vi "Actor Core.vi"(8 "error in (no error)":errorcluster, 11 "Websocket Client Handler in":refnum<class "Websocket Client Handler.lvclass">) -> (0 "error out":errorcluster, 3 "Mediated Asynchronous Actor out":refnum<class "Websocket Client Handler.lvclass">)   [LabVIEW 2016, in "Stream Mediator.lvlib" / "Websocket Client Handler.lvclass"]
doc: "--\nCopyright © 2017 Composed SystemsI All rights reserved.\n\nAuthor: Jon McBee <jon.mcbee@composed.io>\n\nThis library is provided \"AS IS\" ,WITHOUT WARRANTIES OR\nCONDITIONS OF ANY KIND, either express or implied.\n\nComposed Systems -- composed.io\n\nStream 0.0.1.1\nJon McBee - Composed Systems\nCopyright (c) 2017, Composed Systems"
uses:
  <userlib>/Composed Systems/Stream/Mediator/Classes/Websocket Client Handler Actor/Websocket Client Handler/Websocket Client Handler.lvclass
  C:/Program Files (x86)/National Instruments/LabVIEW 2016/user.lib/Composed Systems/Stream/Mediator/Classes/Mediated Asynchronous Actor/Mediated Asynchronous Actor.lvclass
  C:/Program Files (x86)/National Instruments/LabVIEW 2016/user.lib/Composed Systems/Stream/Mediator/Classes/Mediated Actor/Mediated Actor.lvclass
  <userlib>/Composed Systems/Stream/Mediator/Classes/Message Transport Event/Message Transport Event.lvclass
  C:/Program Files (x86)/National Instruments/LabVIEW 2016/user.lib/Composed Systems/Stream/Mediator/Classes/Message Transport Interface/Message Transport Interface.lvclass
  <userlib>/Composed Systems/Stream/Mediator/Classes/Mediated Asynchronous Actor/Mediated Asynchronous Actor.lvclass
  <userlib>/Composed Systems/Stream/Mediator/Classes/Message Broker Interface/Message Broker Interface.lvclass
  <userlib>/Composed Systems/Stream/Mediator/Classes/Websocket Client Handler Actor/Websocket Client Handler Msgs/Write Msg/Write Msg.lvclass
  <userlib>/Composed Systems/Stream/Mediator/Classes/Mediated Actor/Mediated Actor.lvclass
  <userlib>/Composed Systems/Stream/Mediator/Classes/Websocket Client Handler Actor/Websocket Client Handler Msgs/Read Msg/Read Msg.lvclass
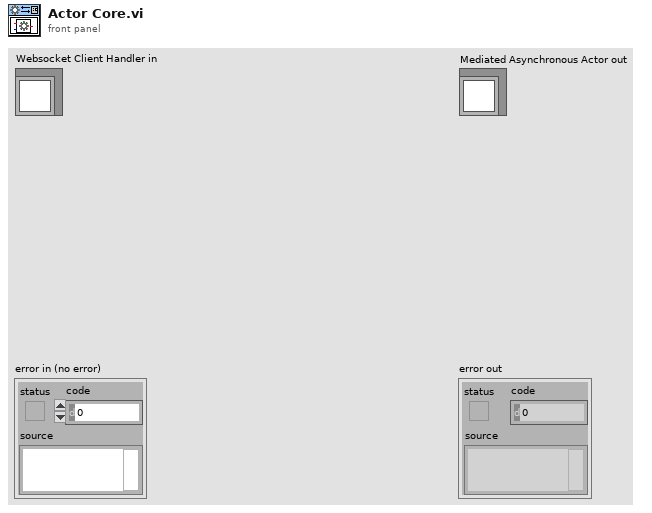
[diagram p1: front panel]
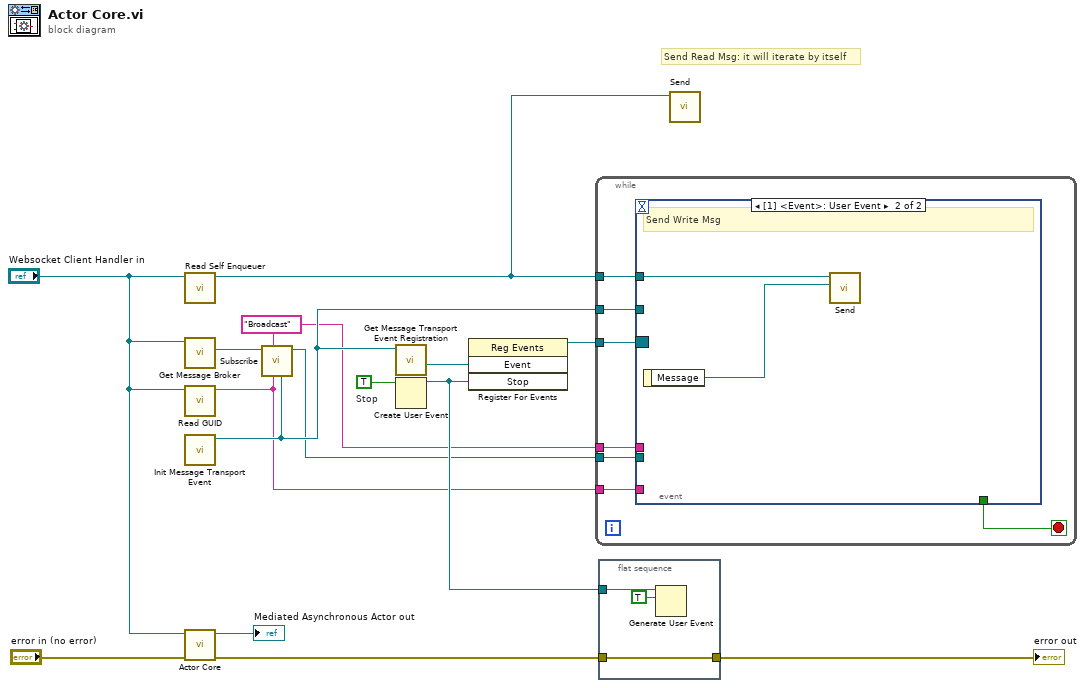
[diagram p0: block diagram]
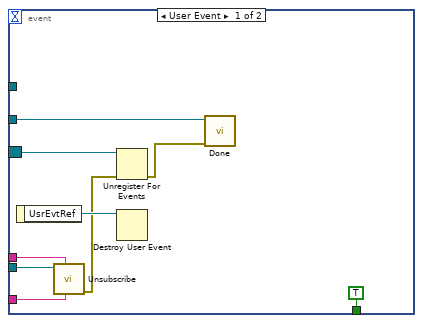
[diagram p2: hidden frame]
diagram:
  w2 = "Broadcast" ("Topic Name")
  w14 = TRUE  # Stop
  # "Send Read Msg: it will iterate by itself"
  n1 = call <userlib>:"Read Self Enqueuer.vi"("Mediated Asynchronous Actor in"="Websocket Client Handler in") -> ("Self Enqueuer"=w1:refnum<class "Message Transport Queue.lvclass">)  [unwired: 10 in]
  n2 = call <userlib>:"Get Message Broker.vi"("Mediated Actor in"="Websocket Client Handler in") -> ("Message Broker"=w6:refnum<class "Message Broker Interface.lvclass">)  [unwired: 9 in, 1 out]
  n3 = call <userlib>:"Read GUID.vi"("Mediated Asynchronous Actor in"="Websocket Client Handler in") -> ("GUID"=w3:string)  [unwired: 10 in]
  n4 = call <userlib>:"Init Message Transport Event.vi"() -> ("Message Transport Event out"=w8:refnum<class "Message Transport Event.lvclass">)  [unwired: 10 in, 1 out]
  n5 = call-parent "Actor Core.vi"("error in (no error)"="error in (no error)", "Mediated Asynchronous Actor in"="Websocket Client Handler in") -> ("error out"=w11:errorcluster, "Mediated Asynchronous Actor out"=→"Mediated Asynchronous Actor out":refnum<class "Websocket Client Handler.lvclass">)  [unwired: 8 in]
  n6 = call-dynamic "Subscribe.vi"("Message Transport Interface"=w8, "Subscriber Name"=w3, "Topic Name"=w2, "Message Broker Interface in"=w6) -> ("Message Broker Interface out"=w4:refnum<class "Message Broker Interface.lvclass">)  [unwired: 5 in, 2 out]
  n7 = call <userlib>:"Get Message Transport Event Registration.vi"("Message Transport Event in"=w8) -> ("Event"=w12:refnum<user-event>)  [unwired: 7 in, 3 out]
  n8 = Create User Event(user event datatype=w14) -> (user event=w9:refnum<user-event>)  [unwired: 1 in, 1 out]
  n9 = register-events(w12, w9) -> (reference out=w13:refnum<event-registration>)  [unwired: 2 in, 1 out]
  n10 = while {
    tunnel: w13 -> [w22]
    tunnel: w8 -> [w20]
    tunnel: w1 -> [w19]
    tunnel: w4 -> [w18]
    tunnel: w3 -> [w17]
    tunnel: w2 -> [w16]
    stop <- w21 stop-if-true
    n11 = event shown="[1] <Event>: User Event" {
      selector: w22 -> [w29 _]
      dyn-events: _ -> [_ _]
      timeout: _ -> [_ _]
      tunnel: [TRUE _] -> w21
      tunnel: w20 -> [w28 _]
      tunnel: w19 -> [_ w33]
      tunnel: w18 -> [w27 _]
      tunnel: w17 -> [w26 _]
      tunnel: w16 -> [w25 _]
      event User Event {
        n12 = event-data() -> ("UsrEvtRef"=w30:refnum<user-event>)  [unwired: 1 in]
        n13 = call-dynamic "Unsubscribe.vi"("Subscriber Name"=w26, "Topic Name"=w25, "Message Broker Interface in"=w27) -> ("error out"=w24:errorcluster)  [unwired: 7 in, 1 out]
        n14 = Unregister For Events(event registration refnum=w29, error in=w24) -> (error out=w23:errorcluster)
        n15 = Destroy User Event(user event=w30) -> ()  [unwired: 1 in, 1 out]
        n16 = call-dynamic "Done.vi"("error in (no error)"=w23, "Message Transport Event in"=w28) -> ()  [unwired: 8 in, 2 out]
      }
      event User Event {
        # "Send Write Msg"
        n17 = event-data() -> ("Message"=w32:refnum<class "Message Interface.lvclass">)  [unwired: 1 in]
        n18 = call <userlib>:"Send.vi"("Message"=w32, "Message Transport Queue"=w33) -> ()  [unwired: 9 in, 1 out]
      }
    }
  }
  n19 = flat-sequence {
    tunnel: w11 -> [w36]
    tunnel: [w36] -> w10
    tunnel: w9 -> [w35]
    frame #0 {
      n20 = Generate User Event(user event=w35, event data cluster=TRUE ("event data")) -> ()  [unwired: 2 in, 2 out]
    }
  }
  n21 = call <userlib>:"Send.vi"("Message Transport Queue"=w1) -> ()  [unwired: 10 in, 1 out]
  "error out" <- w10
